vi "Save_Trav_setup.vi"(0 "Work in Tunnel Coordinates?":T1, 1 "Trav Table":T2[](array[typedef]) {"Carrier_2 Q (l/min)" format="%#.2f"; "Row Duration (mins)" format="%#.1f"; "Row No" min=0; "Trace Gas Concentration (%)" min=0.0 format="%#_4f"; "Carrier_1 Q (l/min)" format="%#.4f"; "Start X" format="%#.2f"; "Start Y" format="%#.2f"; "Start Z" format="%#.2f"; "End X" format="%#.2f"; "End Y" format="%#.2f"; "End Z" format="%#.2f"; "Tunnel Speed" format="%#.2f"; "Averaging time (mins)" min=0.0 format="%#.2f"}, 2 "Fast Plotting?":bool, 4 "Setup filename":path) -> (5 "Trav Table Out":T2[](array[typedef]) {"Carrier_2 Q (l/min)" format="%#.2f"; "Row Duration (mins)" format="%#.1f"; "Row No" min=0; "Trace Gas Concentration (%)" min=0.0 format="%#_4f"; "Carrier_1 Q (l/min)" format="%#.4f"; "Start X" format="%#.2f"; "Start Y" format="%#.2f"; "Start Z" format="%#.2f"; "End X" format="%#.2f"; "End Y" format="%#.2f"; "End Z" format="%#.2f"; "Tunnel Speed" format="%#.2f"; "Averaging time (mins)" min=0.0 format="%#.2f"})   [LabVIEW 2022 SP3]
uses:
  Traverse_cluster.ctl
  Spacing.ctl
  Controls/Multi_run_mode.ctl
  Controls/Tunnel_Coordinates.ctl
  File/Setup_Filetype.ctl
panel:
  # "X           Y          Z"
  # "Start"
  # "End"
  # "X           Y          Z"
  # "Start"
  # "End"
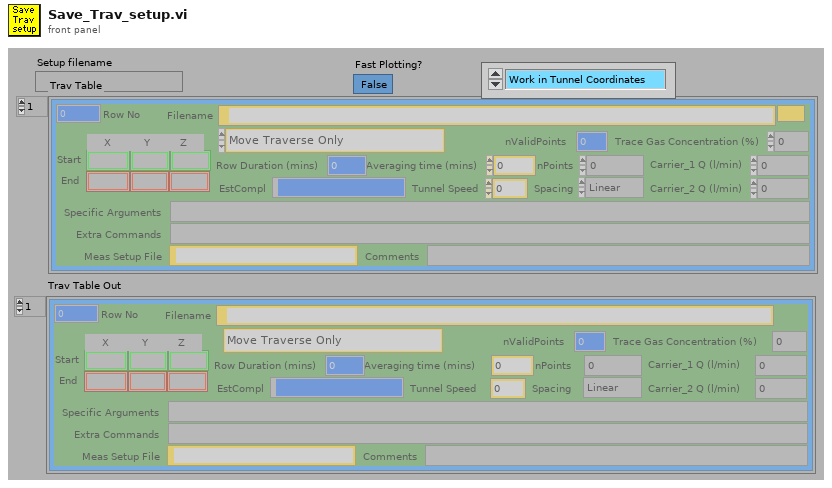
[diagram p1: front panel]
types:
  T1 = typedef "Tunnel_Coordinates.ctl" = enum16{"Work in Tunnel Coordinates", "Work in Model Coordinates"}
  T2 = typedef "Traverse_cluster.ctl" = cluster{"Start X":sgl, "Start Y":sgl, "Start Z":sgl, "End X":sgl, "End Y":sgl, "End Z":sgl, "nPoints":i32, "Spacing":T3, "Filename":path, "Tunnel Speed":dbl, "Averaging time (mins)":dbl, "Extra Commands":string, "Carrier_1 Q (l/min)":dbl, "Carrier_2 Q (l/min)":dbl, "Trace Gas Concentration (%)":dbl, "Specific Arguments":string, "Comments":string, "Row No":i32, "Row Type Selector":T4, "EstCompl":string, "Row Duration (mins)":dbl, "nValidPoints":i32, "Meas Setup File":string}
  T3 = typedef "Spacing.ctl" = enum16{"Linear", "Log", "Gauss", "Specified", "N/A"}
  T4 = typedef "Multi_run_mode.ctl" = enum16{"Move Traverse Only", "Set Tunnel Speed Only", "Set Source Only", "Set Measurement Conditions", "Single Measurement", "Vertical Profile", "Lateral Profile", "Longitudinal Profile", "Multi-Axis Profile", "Explore Volume", "Auto Calibrate", "Meas Fast FID Bkgnd", "Check Beam Power", "Scanning Valve Measurement", "Run VI Named:", "Set ADAM Ch", "Wait (minutes)", "Send Message", "Synchronize With:", "Fall Back to this Row", "Turn Off Row Repeating", "Traverse 3D Volume", "Blank Row", "Jump to Fall Back Row"}
  T5 = enum16{"All Channel Names", "Valid Channel Names"}
  T6 = typedef "Setup_Filetype.ctl" = enum16{"Measurement Setups", "Calibration Setups", "General", "Results File Plotter Setups", "Speed Calib Tweaks"}
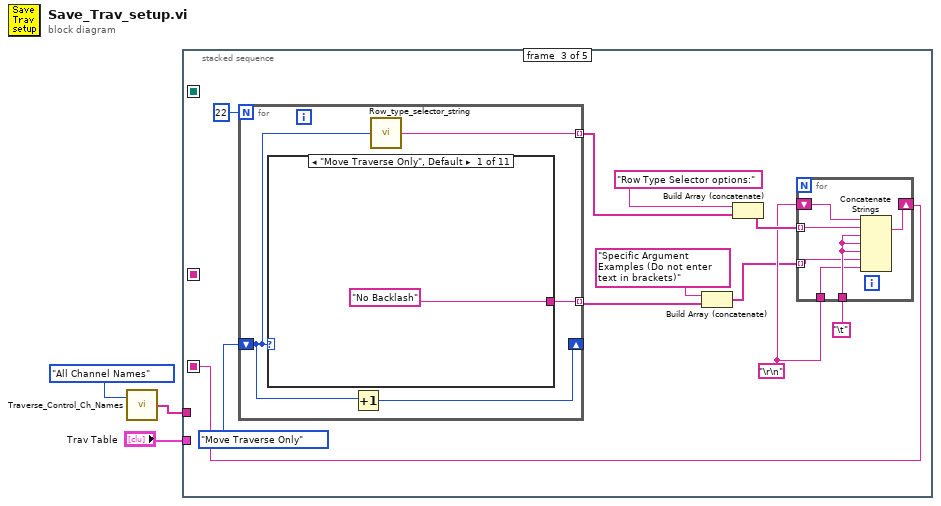
[diagram p0: block diagram]
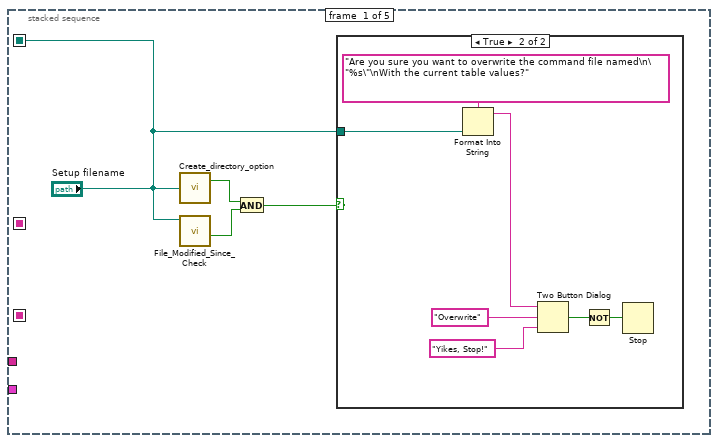
[diagram p2: hidden frame]
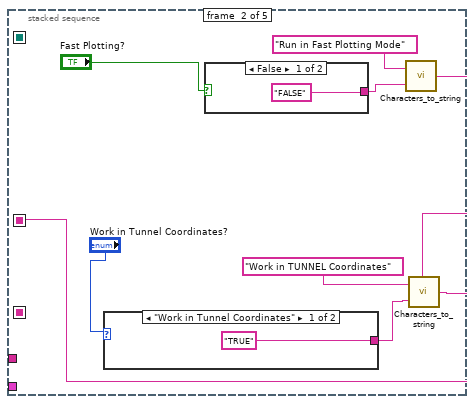
[diagram p4: hidden frame]
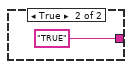
[diagram p5: hidden frame]
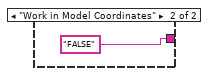
[diagram p6: hidden frame]
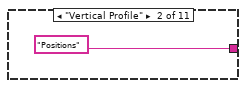
[diagram p7: hidden frame]
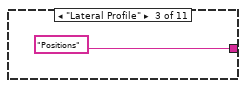
[diagram p8: hidden frame]
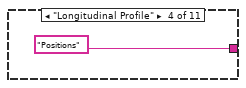
[diagram p9: hidden frame]
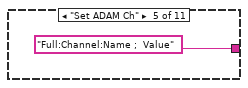
[diagram p10: hidden frame]
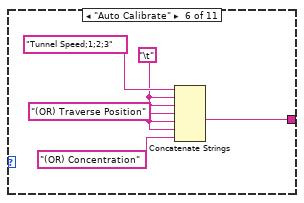
[diagram p11: hidden frame]
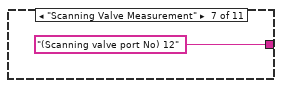
[diagram p12: hidden frame]
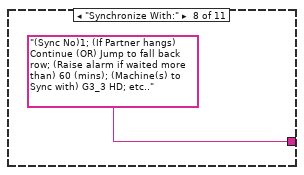
[diagram p13: hidden frame]
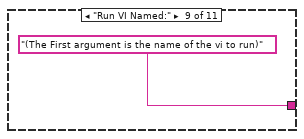
[diagram p14: hidden frame]
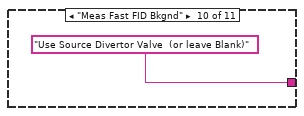
[diagram p15: hidden frame]
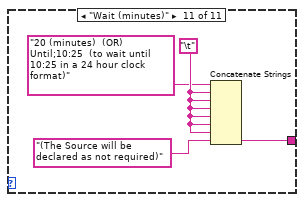
[diagram p16: hidden frame]
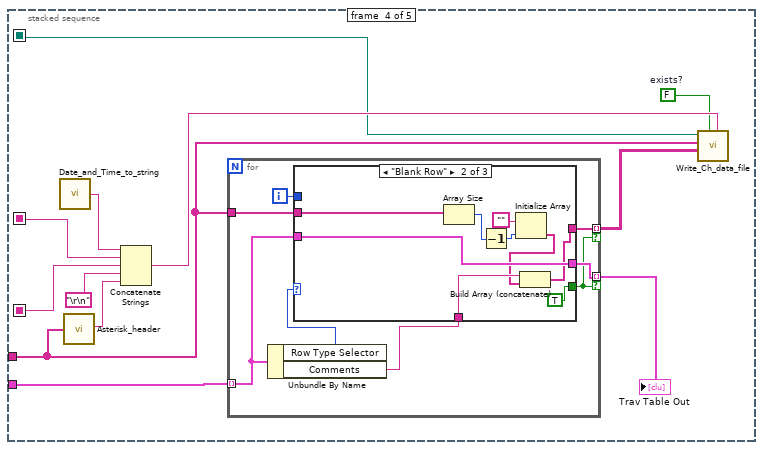
[diagram p17: hidden frame]
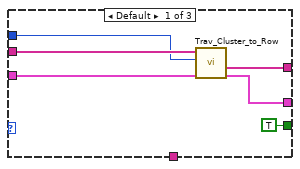
[diagram p18: hidden frame]
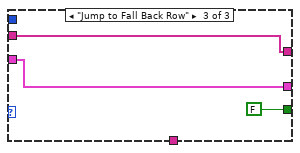
[diagram p19: hidden frame]
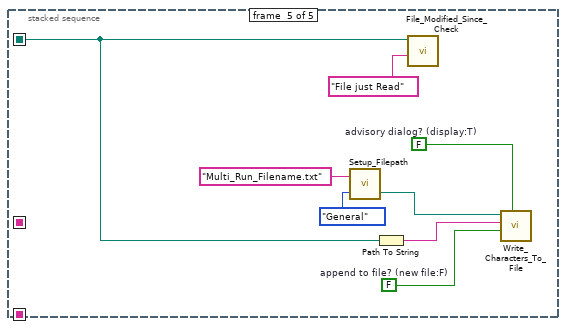
[diagram p20: hidden frame]
diagram:
  n1 = call "Traverse_Control_Ch_Names.vi"("Mode"=T5."All Channel Names") -> ("Channel names"=w3:string[])  [unwired: 1 in]
  n2 = stacked-sequence {
    seq-local: [_ w15 _ _ _] -> [_ _ _ w74 _]
    seq-local: [_ _ w31 _ _] -> [_ _ _ w73 _]
    seq-local: ["Setup filename" _ _ _ _] -> [_ _ _ w67 w105]
    tunnel: w3 -> [_ _ _ w72 _]
    tunnel: "Trav Table" -> [_ _ _ w66 _]
    frame #0 {
      n3 = call "Create_directory_option.vi"("Filename"="Setup filename") -> ("Path is to existing File"=w7:bool)  [unwired: 1 out]
      n4 = call "File_Modified_Since_Check.vi"("File Path"="Setup filename") -> ("modifiedSinceRead"=w4:bool)  [unwired: 7 in, 1 out]
      n5 = And(x=w7, y=w4) -> (x .and. y?=w6:bool)
      n6 = case shown="True" w6 {
        tunnel: "Setup filename" -> [_ w14]
        frame False {
        }
        frame True {
          n7 = Format Into String(format string="Are you sure you want to overwrite the command file named\n\"%s\"\nWith the current table values?" ("Format String"), w14) -> (resulting string=w12:string)  [unwired: 2 in, 1 out]
          n8 = Two Button Dialog(message=w12, 1:"Yikes, Stop!" ("F button name (\"Cancel\")"), 2:"Overwrite" ("T button name (\"OK\")")) -> (T button?=w9:bool)
          n9 = Not(x=w9) -> (.not. x?=w8:bool)
          n10 = Stop(stop? (T)=w8) -> ()
        }
      }
    }
    frame #1 {
      n11 = case shown="\"Work in Tunnel Coordinates\"" "Work in Tunnel Coordinates?" {
        tunnel: ["TRUE" "FALSE" ("f")] -> w20
        frame "Work in Tunnel Coordinates" {
        }
        frame "Work in Model Coordinates" {
        }
      }
      n12 = case shown="False" "Fast Plotting?" {
        tunnel: ["FALSE" ("f") "TRUE"] -> w18
        frame False {
        }
        frame True {
        }
      }
      n13 = call "Characters_to_string.vi"("Characters to write"=w18, "Label for characters"="Run in Fast Plotting Mode") -> ("Output string"=w16:string)  [unwired: 1 in]
      n14 = call "Characters_to_string.vi"("stringIn"=w16, "Characters to write"=w20, "Label for characters"="Work in TUNNEL Coordinates") -> ("Output string"=w15:string)
    }
    frame #2 {
      w36 = "\r\n"
      n15 = for {
        N: 22 -> [_]
        shift-right: [w41] -> _
        shift-left: Multi_run_mode."Move Traverse Only" ("Mode") -> [w40]
        tunnel: [w39] -> w29 mode=indexing
        tunnel: [w38] -> w28 mode=indexing
        n16 = case shown="\"Move Traverse Only\", Default" w40 {
          tunnel: ["No Backlash" "Positions" "Positions" "Positions" "Full:Channel:Name ;  Value" w51 "(Scanning valve port No) 12" "(Sync No)1; (If Partner hangs) Continue (OR) Jump to fall back row; (Raise alarm if waited more than) 60 (mins); (Machine(s) to Sync with) G3_3 HD; etc.." "(The First argument is the name of the vi to run)" "Use Source Divertor Valve  (or leave Blank)" w59] -> w38
          frame "Move Traverse Only", Default {
          }
          frame "Vertical Profile" {
          }
          frame "Lateral Profile" {
          }
          frame "Longitudinal Profile" {
          }
          frame "Set ADAM Ch" {
          }
          frame "Auto Calibrate" {
            w48 = "\t"
            n17 = Concatenate Strings("Tunnel Speed;1;2;3", w48, w48, "(OR) Traverse Position", w48, w48, "(OR) Concentration") -> (w51:string)
          }
          frame "Scanning Valve Measurement" {
          }
          frame "Synchronize With:" {
          }
          frame "Run VI Named:" {
          }
          frame "Meas Fast FID Bkgnd" {
          }
          frame "Wait (minutes)" {
            w57 = "\t"
            n18 = Concatenate Strings("20 (minutes)  (OR) Until;10:25  (to wait until 10:25 in a 24 hour clock format)" ("Substring"), w57, w57, w57, w57, w57, w57, "(The Source will be declared as not required)") -> (w59:string)
          }
        }
        n19 = Increment(x=w40) -> (x+1=w41:T4)
        n20 = call "Row_type_selector_string.vi"("Mode"=w40) -> ("Output string"=w39:string)
      }
      n21 = Build Array (concatenate)("Specific Argument Examples (Do not enter text in brackets)" ("Substring"), w28) -> (w34:string[])
      n22 = Build Array (concatenate)("Row Type Selector options:", w29) -> (w37:string[])
      n23 = for {
        shift-right: [w63] -> w31
        shift-left: w36 -> [w64]
        tunnel: w37 -> [w65] mode=indexing
        tunnel: w36 -> [w60]
        tunnel: w34 -> [w61] mode=indexing
        tunnel: "\t" -> [w62]
        n24 = Concatenate Strings(w64, w65, w62, w62, w62, w61, w60) -> (w63:string)
      }
    }
    frame #3 {
      w76 = FALSE  # exists?
      n25 = call "Date_and_Time_to_string.vi"() -> ("Date and time (spreadsheet)"=w75:string)  [unwired: 4 in, 1 out]
      n26 = call "Asterisk_header.vi"("Channel names"=w72) -> ("Header string"=w68:string)
      n27 = Concatenate Strings(w75, w74, w73, "\r\n", w68) -> (w77:string)
      n28 = for {
        tunnel: w72 -> [w85]
        tunnel: w66 -> [w81] mode=indexing
        tunnel: [w84] -> w71 mode=indexing if=w78
        tunnel: [w83] -> w70 mode=indexing if=w78
        i -> [w82]
        n29 = Unbundle By Name(w81) -> ("Row Type Selector"=w80:T4, "Comments"=w79:string)
        n30 = case shown="\"Blank Row\"" w80 {
          tunnel: w85 -> [w91 w99 w102]
          tunnel: [w90 w93 w102] -> w84
          tunnel: [w89 w100 w103] -> w83
          tunnel: w82 -> [w88 _ _]
          tunnel: w81 -> [w87 w100 w103]
          tunnel: w79 -> [_ w95 _]
          tunnel: [TRUE TRUE FALSE] -> w78
          frame Default {
            n31 = call "Trav_Cluster_to_Row.vi"("Traverse line in"=w87, "Row Number"=w88, "Channel names"=w91) -> ("Traverse line Out"=w89:T2, "Channel Values Out"=w90:string[])  [unwired: 3 out]
          }
          frame "Blank Row" {
            n32 = Array Size(array=w99) -> (size(s)=w97:i32)
            n33 = Decrement(x=w97) -> (x-1=w96:i32)
            n34 = Initialize Array("", w96) -> (w94:string[])
            n35 = Build Array (concatenate)(w95, w94) -> (w93:string[])
          }
          frame "Jump to Fall Back Row" {
          }
        }
      }
      "Trav Table Out" <- w70
      n36 = call "Write_Ch_data_file.vi"("Header string"=w77, "exists?"=w76, "Channel Values"=w71, "Channel names"=w72, "Filename"=w67) -> ()  [unwired: 3 in, 4 out]
    }
    frame #4 {
      w109 = FALSE  # append to file? (new file:F)
      w110 = FALSE  # advisory dialog? (display:T)
      n37 = call "Setup_Filepath.vi"("Setup File Type"=Setup_Filetype."General", "Filename in"="Multi_Run_Filename.txt" ("name or relative path")) -> ("Filename Out"=w106:path)  [unwired: 1 out]
      n38 = Path To String(path=w105) -> (string=w111:string)
      n39 = call "File_Modified_Since_Check.vi"("mode"="File just Read", "File Path"=w105) -> ()  [unwired: 6 in, 2 out]
      n40 = call "Write_Characters_To_File.vi"("file path (dialog if empty)"=w106, "advisory dialog? (display:T)"=w110, "character string"=w111, "append to file? (new file:F)"=w109) -> ()  [unwired: 1 in, 4 out]
    }
  }
